vi "Project Path Getter.vi"(11 "error in (no error)":errorcluster) -> (4 "Path":path, 15 "error out":errorcluster)   [LabVIEW 2021, in "Dictionary.lvlib"]
uses:
  Dictionary.lvlib
  controls/Dictionary States.ctl
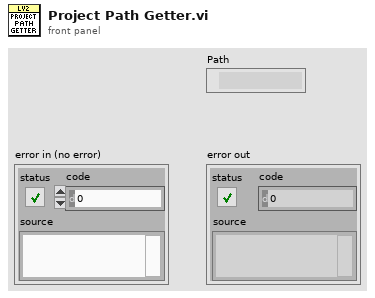
[diagram p1: front panel]
types:
  T1 = typedef "Dictionary.lvlib/Dictionary States.ctl" = enum16{"Set", "Get", "Delete", "Delete All"}
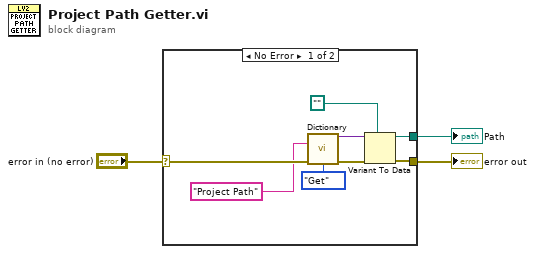
[diagram p0: block diagram]
diagram:
  n1 = case shown="No Error" "error in (no error)" {
    selector: "error in (no error)" -> [w10 w12]
    tunnel: [w6 w12] -> w2
    tunnel: [w4 _] -> w1
    frame No Error {
      n2 = call "Dictionary.vi"("Key"="Project Path", "error in (no error)"=w10, "Dict States"=Dictionary_States."Get") -> ("Variant_Out"=w7:variant, "error out"=w8:errorcluster)  [unwired: 11 in]
      n3 = Variant To Data(error in=w8, type=path "", Variant=w7) -> (data=w4:path, error out=w6:errorcluster)
    }
    frame Error {
    }
  }
  "error out" <- w2
  "Path" <- w1
